vi "sv_Check for Weighting Change (spectrum).vi"(6 "weighting filter":T1 items=["Linear", "A-weighting", "B-weighting", "C-weighting", "ITU-R 468-4", "Dolby", "CCITT", "C-message", "Wb", "Wc", "Wd", "We", "Wf", "Wh", "Wj", "Wk", "Wm", "AES17 20 kHz lowpass", "AES17 40 kHz lowpass", "AES17 20 kHz highpass", "AES17 40 kHz highpass"], 8 "error in (no error)":errorcluster) -> (0 "error out":errorcluster, 1 "weighting has changed":bool, 4 "weighting filter":T1 items=["Linear", "A-weighting", "B-weighting", "C-weighting", "ITU-R 468-4", "Dolby", "CCITT", "C-message", "Wb", "Wc", "Wd", "We", "Wf", "Wh", "Wj", "Wk", "Wm", "AES17 20 kHz lowpass", "AES17 40 kHz lowpass", "AES17 20 kHz highpass", "AES17 40 kHz highpass"])   [LabVIEW 2017]
uses:
  <vilib>/addons/_NISVFA/_Shared subVIs/Controls/svc_Weighting Filter Text Ring.ctl
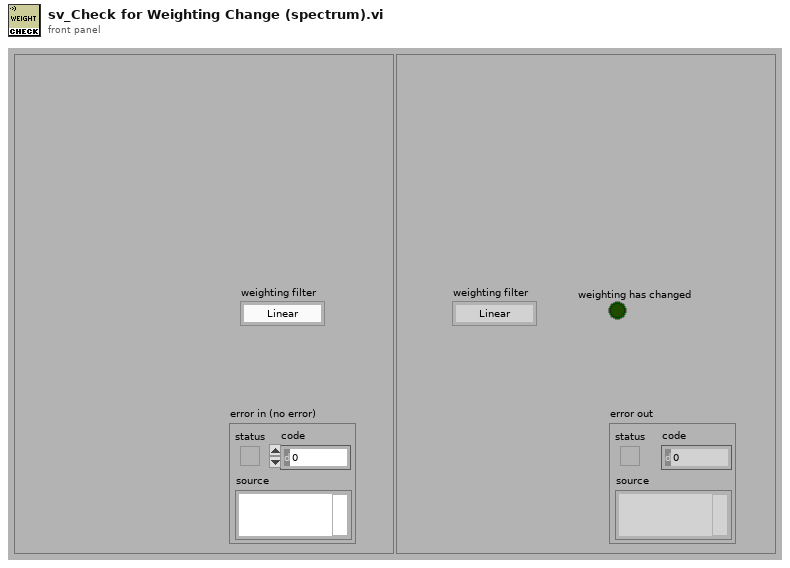
[diagram p1: front panel]
types:
  T1 = typedef "svc_Weighting Filter Text Ring.ctl" = u16
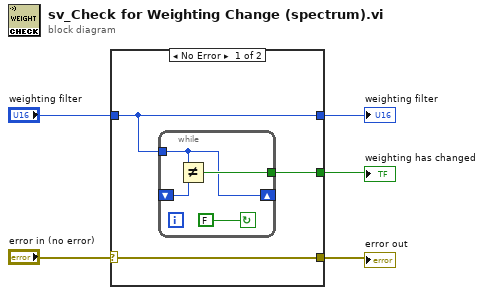
[diagram p0: block diagram]
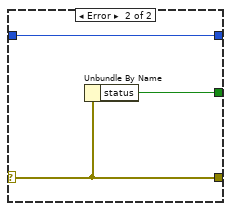
[diagram p2: hidden frame]
diagram:
  n1 = case shown="No Error" "error in (no error)" {
    selector: "error in (no error)" -> [w8 w14]
    tunnel: "weighting filter" -> [w7 w15]
    tunnel: [w8 w14] -> w3
    tunnel: [w7 w15] -> w2
    tunnel: [w6 w13] -> w1
    frame No Error {
      n2 = while {
        tunnel: [w11] -> w6
        tunnel: w7 -> [w9]
        shift-left: _ -> [w10]
        shift-right: [w9] -> _
        stop <- FALSE continue-if-true
        n3 = Not Equal?(x=w9, y=w10) -> (x != y?=w11:bool)
      }
    }
    frame Error {
      n4 = Unbundle By Name(w14) -> ("status"=w13:bool)
    }
  }
  "error out" <- w3
  "weighting filter" <- w2
  "weighting has changed" <- w1
